vi "SiosIfmGetValues.vi"(1 "Device Number":i32) -> (0 "Error":i32)   [LabVIEW 2009]
uses:
  siosifm.dll
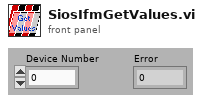
[diagram p1: front panel]
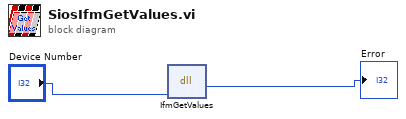
[diagram p0: block diagram]
diagram:
  n1 = dll-call lib="D:/Support/Labview/RE-10/SIOS_IfmDLL/siosifm.dll" fn="IfmGetValues"("devNumber"="Device Number") -> ("Value"=→"Error":i32)  [unwired: 4 in, 2 out]
